vi "Test Compare Different Calls Fail.vi"(8 "error in (no error)":errorcluster, 11 "Test Case In":refnum<class "Tolerant Numeric Comparator Test.lvclass">) -> (0 "error out":errorcluster, 3 "Test Case Out":refnum<class "Tolerant Numeric Comparator Test.lvclass">)   [LabVIEW 2020, in "Tolerant Numeric Comparator Test.lvclass"]
uses:
  Tolerant Numeric Comparator Test.lvclass
  Tolerant Numeric Comparator/Tolerant Numeric Comparator.lvclass
  C:/git/astemes-lmock/sandbox/Comparator/Comparator.lvclass
  Test Interface Mock/Test Interface Mock.lvclass
  C:/git/astemes-lmock/sandbox/Mock/Mock.lvclass
  Tolerant Numeric Comparator Test.lvclass/Tolerant Numeric Comparator Test.ctl
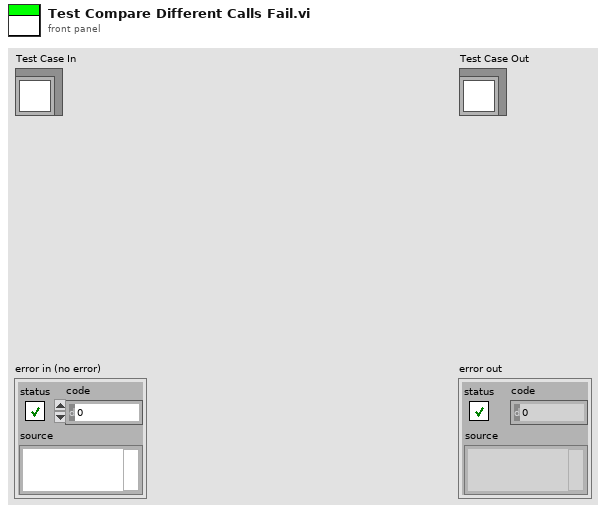
[diagram p1: front panel]
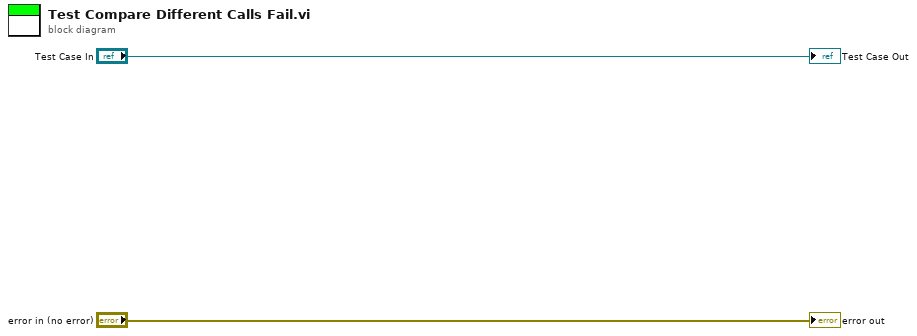
[diagram p0: block diagram]
diagram:
  "error out" <- "error in (no error)"
  "Test Case Out" <- "Test Case In"
